vi "SQL_Table_Test_EndTime_update.vi"(8 "testId":string, 11 "结束时间":string) -> (3 "error out":errorcluster)   [LabVIEW 2014]
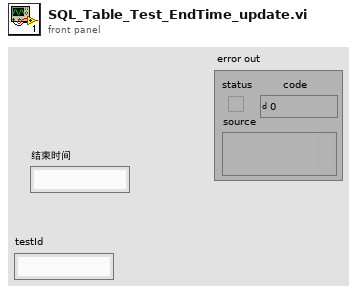
[diagram p1: front panel]
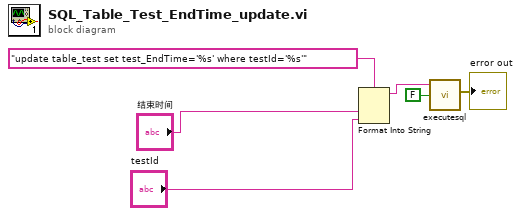
[diagram p0: block diagram]
diagram:
  n1 = Format Into String(format string="update table_test set test_EndTime='%s' where testId='%s'", "结束时间", "testId") -> (resulting string=w3:string)  [unwired: 2 in, 1 out]
  n2 = call "executesql.vi"("Return Data (T)"=FALSE, "Command Text"=w3) -> ("error out"=→"error out":errorcluster)  [unwired: 5 in, 1 out]
